vi "ImageMonoU16ToArray.vi"(8 "error in":errorcluster, 10 "Optional Rectangle":T1, 11 "Image Reference In":T2) -> (0 "error out":errorcluster, 2 "Pixel":u16[][](array[numeric]), 3 "Image Reference Out":T2)   [LabVIEW 2024, in "OpenLvVision_Image.lvlib" / "DataAccess.lvlib"]
doc: "Copies the pixel into an 2D array without an border."
uses:
  DataAccess.lvlib
  Management/TypeDef/Image.ctl
  TypeDef/RectangleI32.ctl
  Management/Management.lvlib
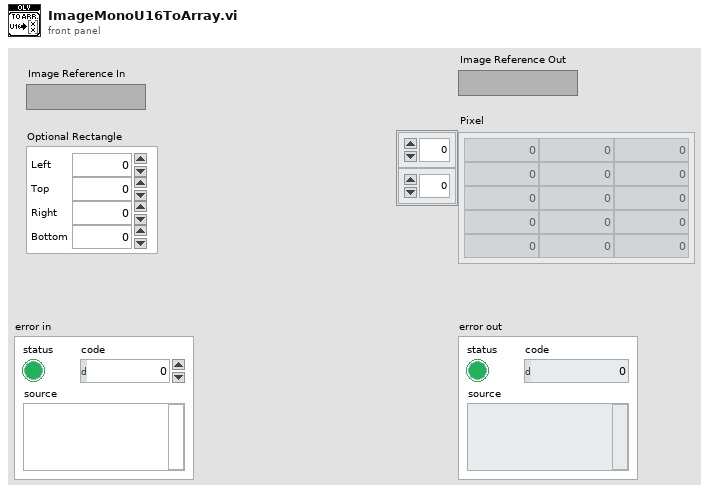
[diagram p1: front panel]
types:
  T1 = typedef "OpenLvVision_Image.lvlib/DataAccess.lvlib/RectangleI32.ctl" = cluster{"Left":i32, "Top":i32, "Right":i32, "Bottom":i32}
  T2 = typedef "OpenLvVision_Image.lvlib/Management.lvlib/Image.ctl" = refnum<image>
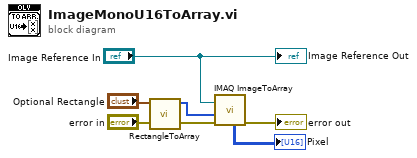
[diagram p0: block diagram]
diagram:
  n1 = call "RectangleToArray.vi"("Optional Rectangle"="Optional Rectangle") -> ("Array"=w2:i32[])  [unwired: 10 in]
  n2 = call "IMAQ ImageToArray"("error in (no error)"="error in", "Optional Rectangle"=w2, "Image"="Image Reference In") -> ("Image Pixels (U16)"=→"Pixel":u16[][], "error out"=→"error out":errorcluster)  [unwired: 1 in, 3 out]
  "Image Reference Out" <- "Image Reference In"
